vi "myRIO__convert__Voltage_to_FPGAvalue.vi"(10 "input_voltage":dbl) -> (1 "output_PortC":i16, 2 "output_PortA":u16)   [LabVIEW 2014]
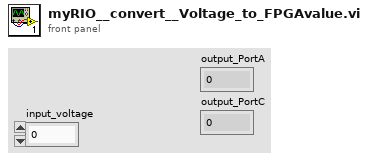
[diagram p1: front panel]
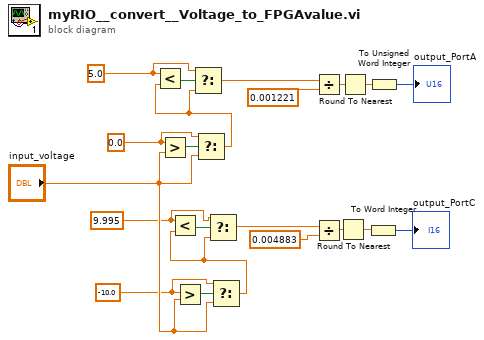
[diagram p0: block diagram]
diagram:
  w13 = -10.0 ("f")
  w7 = 0.0 ("t")
  w8 = 9.995 ("f")
  w14 = 5.0
  n1 = Greater?(x=w7, y="input_voltage") -> (0:w20:bool)
  n2 = Greater?(x=w13, y="input_voltage") -> (0:w17:bool)
  n3 = Select(t=w7, s=w20, f="input_voltage") -> (s? t:f=w19:dbl)
  n4 = Less?(x=w14, y=w19) -> (x < y?=w21:bool)
  n5 = Select(t=w14, s=w21, f=w19) -> (s? t:f=w11:dbl)
  n6 = Select(t=w13, s=w17, f="input_voltage") -> (s? t:f=w16:dbl)
  n7 = Less?(x=w8, y=w16) -> (x < y?=w18:bool)
  n8 = Select(t=w8, s=w18, f=w16) -> (s? t:f=w9:dbl)
  n9 = Divide(x=w11, y=0.001221 ("f")) -> (x/y=w6:dbl)
  n10 = Divide(x=w9, y=0.004883 ("f")) -> (x/y=w4:dbl)
  n11 = Round To Nearest(number=w4) -> (nearest integer value=w3:dbl)
  n12 = Round To Nearest(number=w6) -> (nearest integer value=w5:dbl)
  n13 = To Word Integer(number=w3) -> (16bit integer=→"output_PortC":i16)
  n14 = To Unsigned Word Integer(number=w5) -> (unsigned 16bit integer=→"output_PortA":u16)
